vi "URAPI_Merge.vi"(0 "URAPI False":T1={"Script"="", "Whiles"=[], "Ifs"=[], "Supress Err"=TRUE, "Errors"=""}, 3 "URAPI True":T1={"Script"="", "Whiles"=[], "Ifs"=[], "Supress Err"=TRUE, "Errors"=""}) -> (5 "URAPI Script":T1={"Script"="", "Whiles"=[], "Ifs"=[], "Supress Err"=TRUE, "Errors"=""})   [LabVIEW 2012]
doc: "After a script has been broken into two paths by an if/then statement, it may be rejoined using this VI. If one action is desired regardless of the case statement execution, this VI is to be used."
uses:
  <userlib>/BotSpeak/VIs/Direct/URAPI_Control.ctl
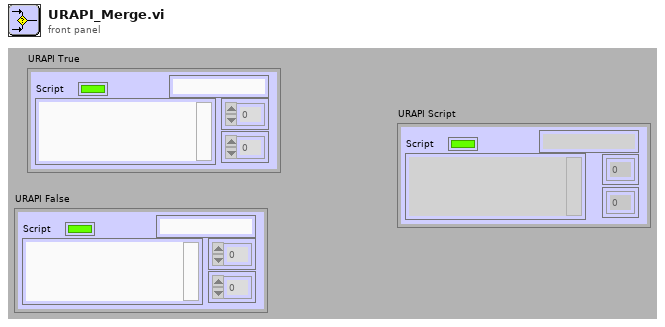
[diagram p1: front panel]
types:
  T1 = typedef "URAPI_Control.ctl" = cluster{"Script":string, "Whiles":u8[], "Ifs":u8[], "Supress Err":bool, "Errors":string}
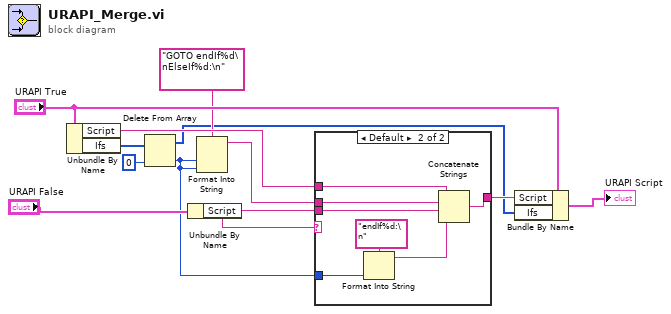
[diagram p0: block diagram]
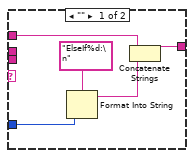
[diagram p2: hidden frame]
diagram:
  n1 = Unbundle By Name("URAPI True") -> ("Script"=w12:string, "Ifs"=w6:u8[])
  n2 = Delete From Array(array=w6, index=0) -> (deleted portion=w2:u8, array with subset deleted=w1:u8[])  [unwired: 1 in]
  n3 = Unbundle By Name("URAPI False") -> ("Script"=w7:string)
  n4 = Format Into String(format string="GOTO endIf%d\nElseIf%d:\n" ("string"), w2, w2) -> (resulting string=w3:string)  [unwired: 2 in, 1 out]
  n5 = case shown="Default" w7 {
    tunnel: w12 -> [w17 w24]
    tunnel: [w16 w23] -> w11
    tunnel: w3 -> [_ w22]
    tunnel: w7 -> [_ w21]
    tunnel: w2 -> [w15 w19]
    frame "" {
      n6 = Format Into String(format string="ElseIf%d:\n" ("string"), w15) -> (resulting string=w13:string)  [unwired: 2 in, 1 out]
      n7 = Concatenate Strings(w17, w13) -> (w16:string)
    }
    frame Default {
      n8 = Format Into String(format string="endIf%d:\n" ("string"), w19) -> (resulting string=w18:string)  [unwired: 2 in, 1 out]
      n9 = Concatenate Strings(w24, w22, w21, w18) -> (w23:string)
    }
  }
  n10 = Bundle By Name(cluster="URAPI True", "Script"=w11, "Ifs"=w1) -> (→"URAPI Script":T1)
